vi "Fpga-Aes-Single-Round.vi"() -> ()   [LabVIEW 2017]
uses:
  <vilib>/Platform/TimedLoop/XDataNode/timing_clust.ctl
  <vilib>/Platform/TimedLoop/XDataNode/nitl_modes.ctl
  <vilib>/Platform/TimedLoop/XDataNode/wakeup.ctl
  <vilib>/rvi/Emulation/niFpgaSctlEmulationGetInTimedLoop.vi
  <vilib>/rvi/Emulation/niFpgaEmulationReportErrorSimple.vi
  <vilib>/rvi/Emulation/niFpgaGetClockAttributes.vi
  <vilib>/rvi/Emulation/niFpgaCriticalErrorInLSC.vi
  <vilib>/Platform/TimedLoop/XDataNode/XDataNode.xnode
  <vilib>/Platform/TimedLoop/XDataNode/XDNodeRunTimeDep.lvlib
panel:
  in  "_a (u8)":u8[](array[numeric])=[112, 140, 87, 5, 26, 105, 60, 215, 234, 195, 31, 158, 103, 201, 83, 249] format="%.0x"
  out "ADD_KEY":u8[](array[numeric])=[34, 130, 200, 79, 19, 60, 180, 37, 0, 203, 98, 21, 244, 242, 162, 212] format="%.0x"
  out "EXP(ADD_KEY)":u8[](array[numeric])=[34, 130, 200, 79, 19, 60, 180, 37, 0, 203, 98, 21, 244, 242, 162, 212] format="%.0x"
  out "EXP(MIX_COLUMNS)":u8[](array[numeric])=[82, 14, 159, 74, 9, 85, 136, 242, 234, 8, 125, 139, 147, 59, 241, 45] format="%.0x"
  out "MIX_COLUMNS":u8[](array[numeric])=[82, 14, 159, 74, 9, 85, 136, 242, 234, 8, 125, 139, 147, 59, 241, 45] format="%.0x"
  out "EXP(SUB_BYTES)":u8[](array[numeric])=[94, 145, 154, 220, 142, 83, 67, 184, 235, 108, 84, 199, 178, 21, 56, 235] format="%.0x"
  out "SUB_BYTES":u8[](array[numeric])=[94, 145, 154, 220, 142, 83, 67, 184, 235, 108, 84, 199, 178, 21, 56, 235] format="%.0x"
  out "SHIFT_ROWS":u8[](array[numeric])=[157, 172, 55, 147, 230, 80, 100, 154, 60, 184, 253, 49, 62, 47, 118, 60] format="%.0x"
  in  "_c (u8)":u8[](array[numeric])=[157, 47, 253, 154, 230, 172, 118, 49, 60, 80, 55, 60, 62, 184, 100, 147] format="%.0x"
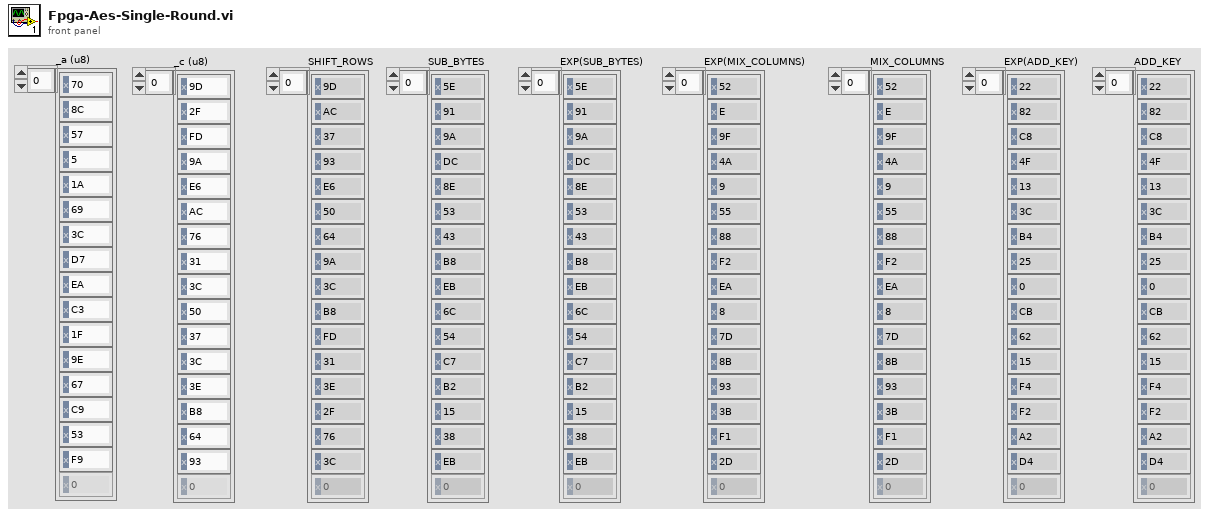
[diagram p1: front panel]
types:
  T1 = typedef "XDNodeRunTimeDep.lvlib/timing_clust.ctl" = cluster{"Expected End [f-1]":u64, "Actual End [f-1]":u64, "Finished Late? [f-1]":bool, "Expected End [i-1]":u64, "Actual End [i-1]":u64, "Finished Late? [i-1]":bool, "Expected Start [i]":u64, "Actual Start [i]":u64, "Expected Start [f]":u64, "Actual Start [f]":u64, "Source Name":string, "Structure Name":string, "Period":i64, "Deadline":i64, "Offset":i64, "Start":i64, "Priority":i32, "Timeout":i32, "Mode":T2, "Wakeup Reason":T3, "Error":errorcluster, "Source Type":string, "Secondary Source Type":string, "Global End Time":u64, "Global Start Time":u64, "Frame Duration":u64, "Iteration Duration":u64, "Assigned CPU":i32, "I/O Scan Engine Mode":u32}
  T2 = typedef "XDNodeRunTimeDep.lvlib/nitl_modes.ctl" = enum32{"No Change", "Process missed periods, maintain original phase", "Discard missed periods, maintain original phase", "Process missed periods, ignore original phase", "Discard missed periods, ignore original phase"}
  T3 = typedef "XDNodeRunTimeDep.lvlib/wakeup.ctl" = enum32{"Normal", "Aborted", "Asynchronous wakeup", "Timing source error", "Timed loop error", "Timeout"}
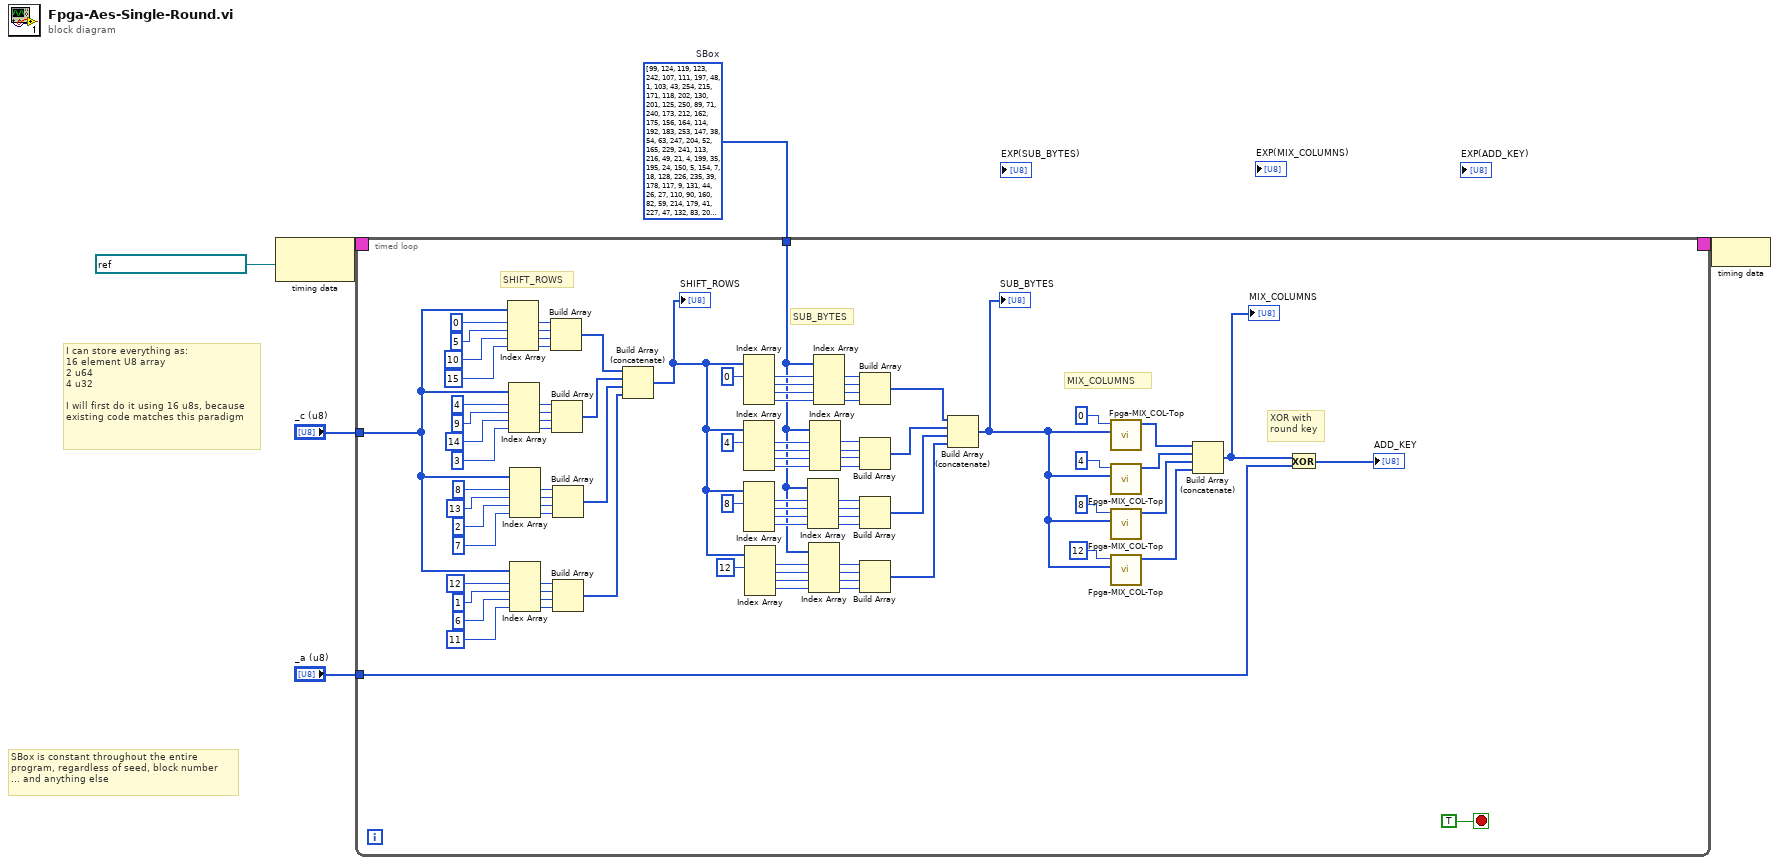
[diagram p0: block diagram]
diagram:
  w5 = u8[] [99, 124, 119, 123, 242, 107, 111, 197, 48, 1, 103, 43, 254, 215, 171, 118, 202, 130, 201, 125, 250, 89, 71, 240, 173, 212, 162, 175, 156, 164, 114, 192, 183, 253, 147, 38, 54, 63, 247, 204, 52, 165, 229, 241, 113, 216, 49, 21, 4, 199, 35, 195, 24, 150, 5, 154, 7, 18, 128, 226, 235, 39, 178, 117, 9, 131, 44, 26, 27, 110, 90, 160, 82, 59, 214, 179, 41, 227, 47, 132, 83, 209, 0, 237, 32, 252, 177, 91, 106, 203, 190, 57, 74, 76, 88, 207, 208, 239, 170, 251, 67, 77, 51, 133, 69, 249, 2, 127, 80, 60, 159, 168, 81, 163, 64, 143, 146, 157, 56, 245, 188, 182, 218, 33, 16, 255, 243, 210, 205, 12, 19, 236, 95, 151, 68, 23, 196, 167, 126, 61, 100, 93, 25, 115, 96, 129, 79, 220, 34, 42, 144, 136, 70, 238, 184, 20, 222, 94, 11, 219, 224, 50, 58, 10, 73, 6, 36, 92, 194, 211, 172, 98, 145, 149, 228, 121, 231, 200, 55, 109, 141, 213, 78, 169, 108, 86, 244, 234, 101, 122, 174, 8, 186, 120, 37, 46, 28, 166, 180, 198, 232, 221, 116, 31, 75, 189, 139, 138, 112, 62, 181, 102, 72, 3, 246, 14, 97, 53, 87, 185, 134, 193, 29, 158, 225, 248, 152, 17, 105, 217, 142, 148, 155, 30, 135, 233, 206, 85, 40, 223, 140, 161, 137, 13, 191, 230, 66, 104, 65, 153, 45, 15, 176, 84, 187, 22]  # SBox
  # "SBox is constant throughout the entire\nprogram, regardless of seed, block number\n... and anything else"
  # "I can store everything as:\n16 element U8 array\n2 u64\n4 u32\n\nI will first do it using 16 u8s, because\nexisting code matches this paradigm"
  n1 = node-c288(refnum<k21> "40 MHz Onboard Clock" ("Source Name")) -> (w4:T1)
  n2 = timed-loop {
    timing: w4 -> [_]
    timing-out: [_] -> w3
    tunnel: "_c (u8)" -> [w66]
    tunnel: w5 -> [w25]
    tunnel: "_a (u8)" -> [w7]
    stop <- TRUE stop-if-true
    # "XOR with\nround key"
    # "MIX_COLUMNS"
    # "SUB_BYTES"
    # "SHIFT_ROWS"
    n3 = Index Array(array=w66, index #1=0 ("index"), index #2=5 ("index"), index #3=10 ("index"), index #4=15 ("index")) -> (element #1=w94:u8, element #2=w93:u8, element #3=w92:u8, element #4=w91:u8)
    n4 = Index Array(array=w66, index #1=4 ("index"), index #2=9 ("index"), index #3=14 ("index"), index #4=3 ("index")) -> (element #1=w62:u8, element #2=w86:u8, element #3=w85:u8, element #4=w84:u8)
    n5 = Index Array(array=w66, index #1=8 ("index"), index #2=13 ("index"), index #3=2 ("index"), index #4=7 ("index")) -> (element #1=w63:u8, element #2=w80:u8, element #3=w79:u8, element #4=w78:u8)
    n6 = Index Array(array=w66, index #1=12 ("index"), index #2=1 ("index"), index #3=6 ("index"), index #4=11 ("index")) -> (element #1=w64:u8, element #2=w74:u8, element #3=w73:u8, element #4=w72:u8)
    n7 = Build Array(w94, w93, w92, w91) -> (w90:u8[])
    n8 = Build Array(w62, w86, w85, w84) -> (w71:u8[])
    n9 = Build Array(w63, w80, w79, w78) -> (w70:u8[])
    n10 = Build Array(w64, w74, w73, w72) -> (w65:u8[])
    n11 = Build Array (concatenate)(w90, w71, w70, w65) -> (w36:u8[])
    "SHIFT_ROWS" <- w36
    n12 = Index Array(array=w36, index #1=0 ("index")) -> (element #1=w59:u8, element #2=w58:u8, element #3=w57:u8, element #4=w56:u8)  [unwired: 3 in]
    n13 = Index Array(array=w36, index #1=4 ("index")) -> (element #1=w45:u8, element #2=w44:u8, element #3=w43:u8, element #4=w42:u8)  [unwired: 3 in]
    n14 = Index Array(array=w36, index #1=8 ("index")) -> (element #1=w49:u8, element #2=w48:u8, element #3=w47:u8, element #4=w46:u8)  [unwired: 3 in]
    n15 = Index Array(array=w36, index #1=12 ("index")) -> (element #1=w40:u8, element #2=w39:u8, element #3=w38:u8, element #4=w37:u8)  [unwired: 3 in]
    n16 = Index Array(array=w25, index #1=w49, index #2=w48, index #3=w47, index #4=w46) -> (element #1=w31:u8, element #2=w28:u8, element #3=w30:u8, element #4=w29:u8)
    n17 = Index Array(array=w25, index #1=w40, index #2=w39, index #3=w38, index #4=w37) -> (element #1=w23:u8, element #2=w24:u8, element #3=w26:u8, element #4=w27:u8)
    n18 = Index Array(array=w25, index #1=w45, index #2=w44, index #3=w43, index #4=w42) -> (element #1=w32:u8, element #2=w33:u8, element #3=w34:u8, element #4=w35:u8)
    n19 = Index Array(array=w25, index #1=w59, index #2=w58, index #3=w57, index #4=w56) -> (element #1=w55:u8, element #2=w54:u8, element #3=w53:u8, element #4=w52:u8)
    n20 = Build Array(w55, w54, w53, w52) -> (w61:u8[])
    n21 = Build Array(w32, w33, w34, w35) -> (w22:u8[])
    n22 = Build Array(w31, w28, w30, w29) -> (w21:u8[])
    n23 = Build Array(w23, w24, w26, w27) -> (w20:u8[])
    n24 = Build Array (concatenate)(w61, w22, w21, w20) -> (w13:u8[])
    "SUB_BYTES" <- w13
    n25 = call "Fpga-MIX_COL-Top.vi"("Array in"=w13, "index"=0) -> ("Array out"=w17:u8[])  [unwired: 9 in]
    n26 = call "Fpga-MIX_COL-Top.vi"("Array in"=w13, "index"=4) -> ("Array out"=w12:u8[])  [unwired: 9 in]
    n27 = call "Fpga-MIX_COL-Top.vi"("Array in"=w13, "index"=8) -> ("Array out"=w11:u8[])  [unwired: 9 in]
    n28 = call "Fpga-MIX_COL-Top.vi"("Array in"=w13, "index"=12) -> ("Array out"=w10:u8[])  [unwired: 9 in]
    n29 = Build Array (concatenate)(w17, w12, w11, w10) -> (w8:u8[])
    "MIX_COLUMNS" <- w8
    n30 = Exclusive Or(1:w7, 2:w8) -> (0:→"ADD_KEY":u8[])
  }
  n31 = node-c288(w3) -> ()
